vi "Set Temperature.vi"(4 "Channel":i32, 8 "error in (no error)":errorcluster, 9 "Rate (K/min)":dbl, 10 "Temperature (K)":dbl, 11 "Instrument.Oxford1820 in":refnum<class "Instrument.Oxford1820.lvclass">) -> (0 "error out":errorcluster, 3 "Instrument.Oxford1820 out":refnum<class "Instrument.Oxford1820.lvclass">)   [LabVIEW 2016, in "Instrument.Oxford1820.lvclass"]
uses:
  Instrument.Oxford1820.lvclass
  <userlib>/LevyLab/Levylab Instruments/Instrument Types/Cryostat/Instrument.Cryostat.lvclass
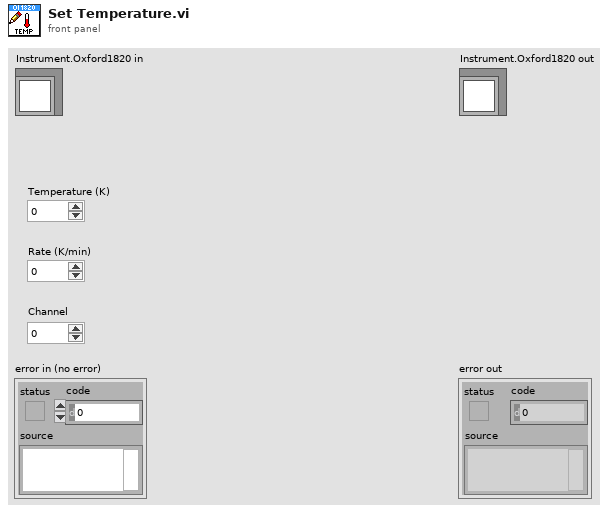
[diagram p1: front panel]
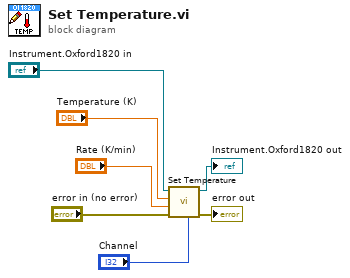
[diagram p0: block diagram]
diagram:
  n1 = call-parent "Set Temperature.vi"("Channel"="Channel", "error in (no error)"="error in (no error)", "Rate (K/min)"="Rate (K/min)", "Temperature (K)"="Temperature (K)", "Instrument.Cryostat in"="Instrument.Oxford1820 in") -> ("error out"=→"error out":errorcluster, "Instrument.Cryostat out"=→"Instrument.Oxford1820 out":refnum<class "Instrument.Oxford1820.lvclass">)  [unwired: 5 in]
